vi "OdomLaserSubscriber.vi"() -> (0 "Odom Error Out":errorcluster)   [LabVIEW 2016]
doc: "Reads in the odometry from the Turtlebot"
uses:
  <vilib>/Tufts CEEO ROS for LabVIEW Software/ROS/Code/SubVIs/_ROSDirection.ctl
  <vilib>/Tufts CEEO ROS for LabVIEW Software/ROS/Code/Console/Servers/ServerSubs/TopicDef.ctl
panel:
  in  "Max Odom Pts":dbl=500.0
  out "Scan Details":T1={"Min. Angle (rad)"=-2.3561899662017822, "Max. Angle (rad)"=2.3561899662017822, "Angle Incr. (rad)"=0.006554075051099062, "Time Inc. (s)"=0.0, "Scan Time (s)"=0.0, "Min. Range (m)"=0.10000000149011612, "Max. Range (m)"=1.0089348943138683e-42}
  in  "Clear Plot":bool
  in  "Update Time (ms)":u32=300
  out "Laser Scan Plot (in Husky Frame)":cluster{dbl[], dbl[]}(graph)
  out "Scan Error Out":errorcluster
  out "2D Pose":cluster{"x":dbl, "y":dbl}={"x"=2.1588546690121686, "y"=0.6824320147682317}
  out "Husky Pose Plot":cluster{"X":dbl, "Y":dbl}[](graph)=[{"X"=2.1588546690121686, "Y"=0.6824320147682317}]
  out "Husky EKF Odometry":T2={"PoseCovariance"={"Pose"={"Position\n(xyz)"={"x"=2.1588546690121686, "y"=0.6824320147682317, "z"=0.0}, "Orientation\n(Quaternions)"={"x"=0.0, "y"=0.0, "z"=-0.6154075833582808, "w"=0.7882090499005455}}, "Covariance[1,1]"=150.49515067805697}}
  in  "Stop Subscribing":bool
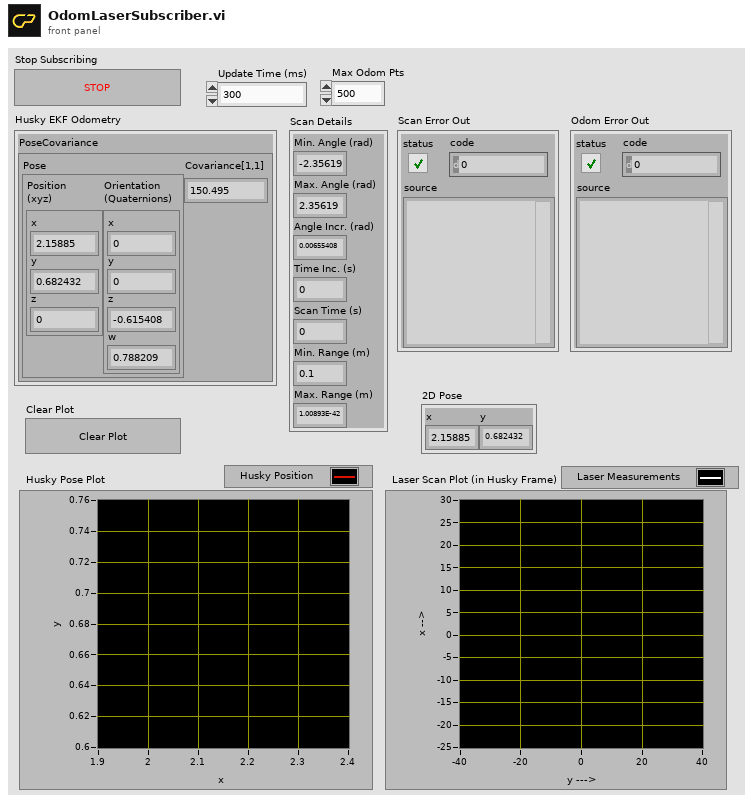
[diagram p1: front panel]
types:
  T1 = cluster{"Min. Angle (rad)":dbl, "Max. Angle (rad)":dbl, "Angle Incr. (rad)":dbl, "Time Inc. (s)":dbl, "Scan Time (s)":dbl, "Min. Range (m)":dbl, "Max. Range (m)":dbl}
  T2 = cluster{"PoseCovariance":cluster{"Pose":cluster{"Position\n(xyz)":cluster{"x":dbl, "y":dbl, "z":dbl}, "Orientation\n(Quaternions)":cluster{"x":dbl, "y":dbl, "z":dbl, "w":dbl}}, "Covariance[1,1]":dbl}}
  T3 = typedef "TopicDef.ctl" = cluster{"Topic":string, "Type":string, "Action":T4, "Update (ms)":u16, "queue size":u16}
  T4 = typedef "_ROSDirection.ctl" = enum16{"Node", "Publisher", "Subscriber", "ServiceClient", "ServiceProvider"}
  T5 = typedef "_ROSControl.ctl" = cluster{"topic port":u16, "Node":string, "topic":string, "type":string, "node port":u16, "error ":errorcluster, "Direction":T4, "Update (ms)":u16, "FIFO size":u16}
  T6 = cluster{"PoseCovariance":cluster{"Pose":cluster{"Point":cluster{"x":dbl, "y":dbl, "z":dbl}, "Quaternion":cluster{"x":dbl, "y":dbl, "z":dbl, "w":dbl}}, "Covariance":dbl}}
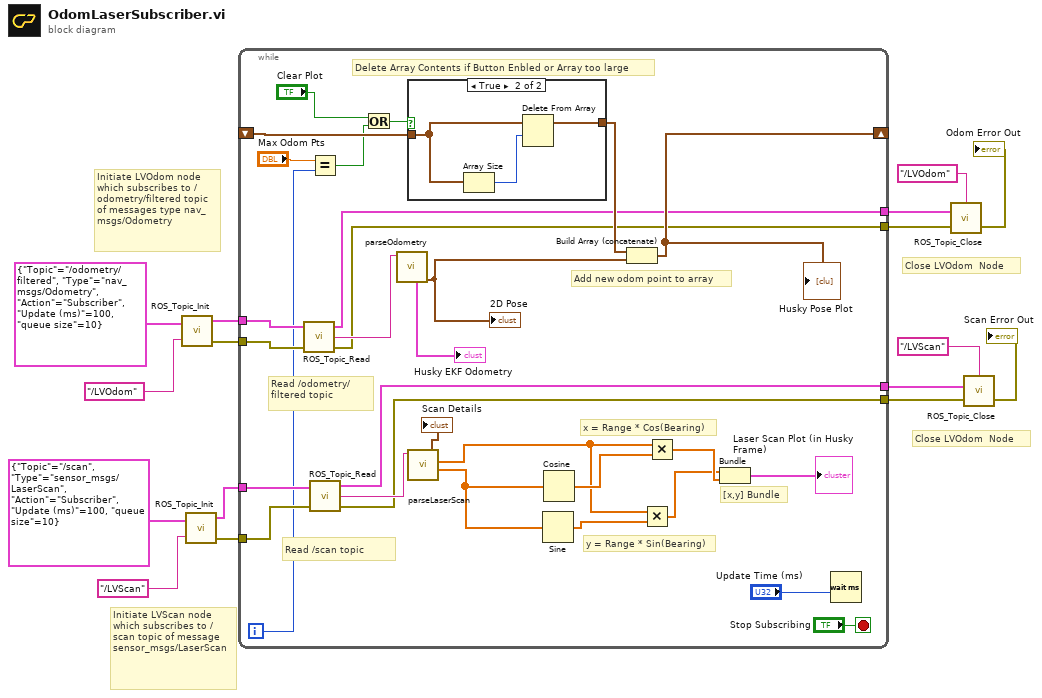
[diagram p0: block diagram]
diagram:
  # "Close LVOdom  Node"
  # "Close LVOdom  Node"
  # "Initiate LVScan node which subscribes to /scan topic of message sensor_msgs/LaserScan"
  # "Initiate LVOdom node which subscribes to /odometry/filtered topic of messages type nav_msgs/Odometry"
  n1 = call <vilib>:"ROS_Topic_Init.vi"("Definitions"=T3 {"Topic"="/odometry/filtered", "Type"="nav_msgs/Odometry", "Action"=enum."Subscriber", "Update (ms)"=100, "queue size"=10}, "node"="/LVOdom") -> ("ROS out"=w12:T5, "error out"=w11:errorcluster)  [unwired: 1 in]
  n2 = call <vilib>:"ROS_Topic_Init.vi"("Definitions"=T3 {"Topic"="/scan", "Type"="sensor_msgs/LaserScan", "Action"=enum."Subscriber", "Update (ms)"=100, "queue size"=10}, "node"="/LVScan") -> ("ROS out"=w10:T5, "error out"=w9:errorcluster)  [unwired: 1 in]
  n3 = while {
    shift-right: [w45] -> _
    shift-left: _ -> [w31]
    tunnel: w12 -> [w36]
    tunnel: w11 -> [w35]
    tunnel: w10 -> [w34]
    tunnel: w9 -> [w33]
    tunnel: [w28] -> w8
    tunnel: [w27] -> w7
    tunnel: [w26] -> w5
    tunnel: [w25] -> w3
    i -> [w18]
    stop <- "Stop Subscribing" stop-if-true
    # "Add new odom point to array"
    # "Read /scan topic"
    # "Read /odometry/filtered topic"
    # "Delete Array Contents if Button Enbled or Array too large"
    # "[x,y] Bundle"
    # "y = Range * Sin(Bearing)"
    # "x = Range * Cos(Bearing)"
    n4 = call <vilib>:"ROS_Topic_Read.vi"("error in (no error)"=w35, "ROS in"=w36) -> ("error out"=w25:errorcluster, "Reply"=w44:string, "ROS out"=w27:T5)  [unwired: 1 in]
    n5 = Equal?(x="Max Odom Pts", y=w18) -> (x = y?=w17:bool)
    n6 = call <vilib>:"ROS_Topic_Read.vi"("error in (no error)"=w33, "ROS in"=w34) -> ("error out"=w26:errorcluster, "Reply"=w41:string, "ROS out"=w28:T5)  [unwired: 1 in]
    n7 = Or(x="Clear Plot", y=w17) -> (x .or. y?=w20:bool)
    n8 = call "parseOdometry.vi"("msg in"=w44) -> ("Odometry"=→"Husky EKF Odometry":T6, "Pose 2D"=w42:cluster{"x":dbl, "y":dbl})  [unwired: 3 in, 3 out]
    "2D Pose" <- w42
    n9 = case shown="True" w20 {
      tunnel: [w47 w49] -> w30
      tunnel: w31 -> [w47 w48]
      frame False {
      }
      frame True {
        n10 = Array Size(array=w48) -> (size(s)=w50:i32)
        n11 = Delete From Array "Delete From Array"(array=w48, length=w50) -> (array with subset deleted=w49:cluster{"x":dbl, "y":dbl}[])  [unwired: 1 in, 1 out]
      }
    }
    n12 = call "parseLaserScan.vi"("msg in"=w41) -> ("Bearing Array"=w39:dbl[], "Range Array"=w38:sgl[], "Scan Details"=→"Scan Details":T1)  [unwired: 3 in, 1 out]
    n13 = Sine(x=w39) -> (sin(x)=w37:dbl[])
    n14 = Cosine(x=w39) -> (cos(x)=w40:dbl[])
    n15 = Build Array (concatenate)(w30, w42) -> (w45:cluster{"x":dbl, "y":dbl}[])
    "Husky Pose Plot" <- w45
    n16 = Multiply(x=w38, y=w37) -> (x*y=w23:dbl[])
    n17 = Multiply(x=w38, y=w40) -> (x*y=w24:dbl[])
    n18 = Bundle(w23, w24) -> (→"Laser Scan Plot (in Husky Frame)":cluster{dbl[], dbl[]})  [unwired: 1 in]
    n19 = Wait (ms)(milliseconds to wait="Update Time (ms)") -> ()  [unwired: 1 out]
  }
  n20 = call <vilib>:"ROS_Topic_Close.vi"("error in"=w3, "ROS in"=w7, "node"="/LVOdom") -> ("error out"=→"Odom Error Out":errorcluster)  [unwired: 1 in]
  n21 = call <vilib>:"ROS_Topic_Close.vi"("error in"=w5, "ROS in"=w8, "node"="/LVScan") -> ("error out"=→"Scan Error Out":errorcluster)  [unwired: 1 in]
